vi "Subvi in range.vi"(8 "Max":u64, 9 "Input":u64, 10 "Min":u64) -> (1 "In range":bool)   [LabVIEW 2017]
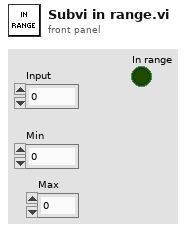
[diagram p1: front panel]
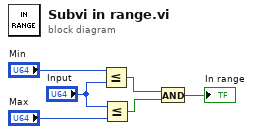
[diagram p0: block diagram]
diagram:
  n1 = Less Or Equal?(x="Min", y="Input") -> (x <= y?=w3:bool)
  n2 = Less Or Equal?(x="Input", y="Max") -> (x <= y?=w2:bool)
  n3 = And(x=w3, y=w2) -> (x .and. y?=→"In range":bool)
